vi "setup_oscillators.vi"(8 "error in (no error)":errorcluster, 11 "Handle In":T1 {"Handle" format="0x%08x"; "Conn" format="0x%08x"}) -> (0 "error out":errorcluster, 3 "Handle Out":T1 {"Handle" format="0x%08x"; "Conn" format="0x%08x"})   [LabVIEW 2019]
uses:
  Equipment/Zurich Instruments LabOne/Public/ziTypeHandle.ctl
  Instrument_Setup.vi
  Equipment/Zurich Instruments LabOne/Public/Configure/ziSetValueDouble.vi
  Equipment/Zurich Instruments LabOne/Zurich Instruments LabOne.lvlib
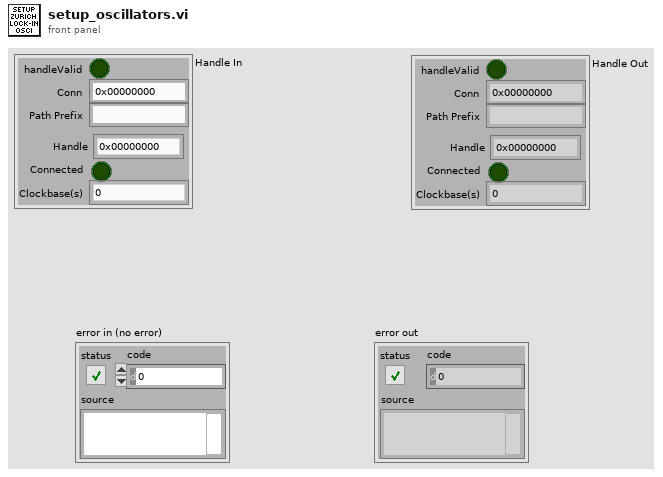
[diagram p1: front panel]
types:
  T1 = typedef "Zurich Instruments LabOne.lvlib/ziTypeHandle.ctl" = cluster{"handleValid":bool, "Conn":u64, "Path Prefix":string, "Handle":u64, "Connected":bool, "Clockbase(s)":dbl}
  T2 = typedef "Control 3.ctl" = cluster{"Adress":string, "Load Settings from File":bool, "Output_Demod1":enum16{"Aux 1", "Aux 2", "Aux 3", "Aux 4"}, "Input_Demod1":enum16{"Sig In 1", "Curr In 1", "Trigger 1", "Trigger 2", "Aux Out 1", "Aux Out 2", "Aux Out 3", "Aux Out 4", "Aux In 1", "Aux In 2", "Constant"}, "Input_Mode_Demod1":enum16{"single ended", "differential"}, "Bandwith_Mode_Demod1":enum16{"TC", "BW NEP", "BW 3dB"}, "Bandw_Value_demod1":dbl, "Demod1_Range":dbl, "Demod1_Harmonic":dbl, "Trigger_Demod1":enum16{"Manual", "External"}, "osc1_freq":dbl, "osc1_amp":dbl, "Demod1_scaling":dbl, "osc2_freq":dbl, "osc2_amp":dbl, "osc3_freq":dbl, "osc3_amp":dbl, "osc4_freq":dbl, "osc4_amp":dbl, "Demod1_Phase (deg)":dbl, "Demod1_order":ext, "Demod1_coupling":enum16{"DC", "AC"}, "Demod1_shields":enum16{"Ground", "Float"}, "Demod1_input_resistance":enum16{"10M", "50"}, "Demod1_Ref_oscillator":ext, "Demod1_output_imp":enum16{"Disable", "Enable"}, "Demod1_output_diff":enum16{"Disable", "Enable"}, "Demod1_rate":dbl, "Demod1_Output_range":dbl, "Output_Demod2":enum16{"Aux 1", "Aux 2", "Aux 3", "Aux 4"}, "Demod2_input":enum16{"Sig In 1", "Curr In 1", "Trigger 1", "Trigger 2", "Aux Out 1", "Aux Out 2", "Aux Out 3", "Aux Out 4", "Aux In 1", "Aux In 2", "Constant"}, "Input_Mode_Demod2":enum16{"single ended", "differential"}, "Bandwith_Mode_Demod2":enum16{"TC", "BW NEP", "BW 3dB"}, "Bandw_Value_demod2":dbl, "Demod2_Range":dbl, "Demod2_Harmonic":dbl, "Trigger_Demod2":enum16{"Manual", "External"}, "Demod2_scaling":dbl, "Demod2_Phase (deg)":dbl, "Demod2_order":ext, "Demod2_coupling":enum16{"DC", "AC"}, "Demod2_shields":enum16{"Ground", "Float"}, "Demod2_input_resistance":enum16{"10M", "50"}, "Demod2_Ref_oscillator":ext, "Demod2_output_imp":enum16{"Disable", "Enable"}, "Demod2_output_diff":enum16{"Disable", "Enable"}, "Demod2_rate":dbl, "Demod2_Output_range":dbl, "Output_Demod3":enum16{"Aux 1", "Aux 2", "Aux 3", "Aux 4"}, "Demod3_input":enum16{"Sig In 1", "Curr In 1", "Trigger 1", "Trigger 2", "Aux Out 1", "Aux Out 2", "Aux Out 3", "Aux Out 4", "Aux In 1", "Aux In 2", "Constant"}, "Input_Mode_Demod3":enum16{"single ended", "differential"}, "Bandwith_Mode_Demod2":enum16{"TC", "BW NEP", "BW 3dB"}, "Bandw_Value_demod3":dbl, "Demod3_Range":dbl, "Demod3_Harmonic":dbl, "Trigger_Demod3":enum16{"Manual", "External"}, "Demod3_scaling":dbl, "Demod3_Phase (deg)":dbl, "Demod3_order":ext, "Demod3_coupling":enum16{"DC", "AC"}, "Demod3_shields":enum16{"Ground", "Float"}, "Demod3_input_resistance":enum16{"10M", "50"}, "Demod3_Ref_oscillator":ext, "Demod3_output_imp":enum16{"Disable", "Enable"}, "Demod3_output_diff":enum16{"Disable", "Enable"}, "Demod3_rate":dbl, "Demod3_Output_range":dbl, "Output_Demod4":enum16{"Aux 1", "Aux 2", "Aux 3", "Aux 4"}, "Demod4_input":enum16{"Sig In 1", "Curr In 1", "Trigger 1", "Trigger 2", "Aux Out 1", "Aux Out 2", "Aux Out 3", "Aux Out 4", "Aux In 1", "Aux In 2", "Constant"}, "Input_Mode_Demod4":enum16{"single ended", "differential"}, "Bandwith_Mode_Demod4":enum16{"TC", "BW NEP", "BW 3dB"}, "Bandw_Value_demod4":dbl, "Demod4_Range":dbl, "Demod4_Harmonic":dbl, "Trigger_Demod4":enum16{"Manual", "External"}, "Demod4_scaling":dbl, "Demod4_Phase (deg)":dbl, "Demod4_order":ext, "Demod4_coupling":enum16{"DC", "AC"}, "Demod4_shields":enum16{"Ground", "Float"}, "Demod4_input_resistance":enum16{"10M", "50"}, "Demod4_Ref_oscillator":ext, "Demod4_output_imp":enum16{"Disable", "Enable"}, "Demod4_output_diff":enum16{"Disable", "Enable"}, "Demod4_rate":dbl, "Demod4_Output_range":dbl, "Oscillator1_Amp_units":enum16{"Vpk", "Vrms", "VdBm"}, "Oscillator4_Amp_units":enum16{"Vpk", "Vrms", "VdBm"}, "Oscillator2_Amp_units":enum16{"Vpk", "Vrms", "VdBm"}, "Oscillator3_Amp_units":enum16{"Vpk", "Vrms", "VdBm"}, "Demod1_sync_filter":enum16{"Disable", "Enable"}, "Demod 1 (on/off)":bool, "Demod 2 (on/off) ":bool, "Demod 3 (on/off) ":bool, "Demod 4 (on/off) ":bool, " Sigouts 1 (on/off)":bool, " Sigouts 2 (on/off) ":bool, " Sigouts 3 (on/off)":bool, " Sigouts 4 (on/off) ":bool, "Demod2_sync_filter":enum16{"Disable", "Enable"}, "Demod1_auto_outp_rang":enum16{"Disable", "Enable"}, "Demod2_auto_outp_rang ":enum16{"Disable", "Enable"}}
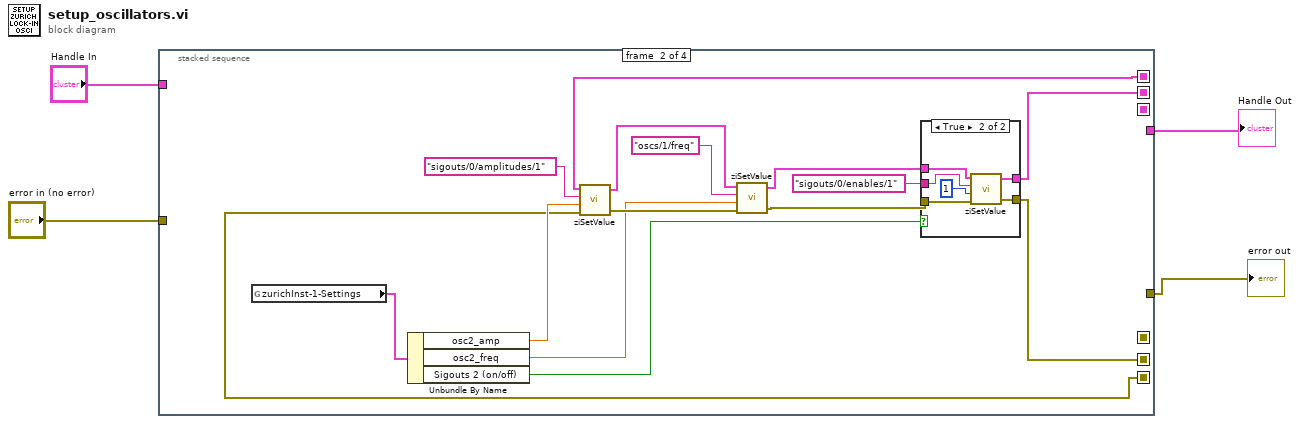
[diagram p0: block diagram]
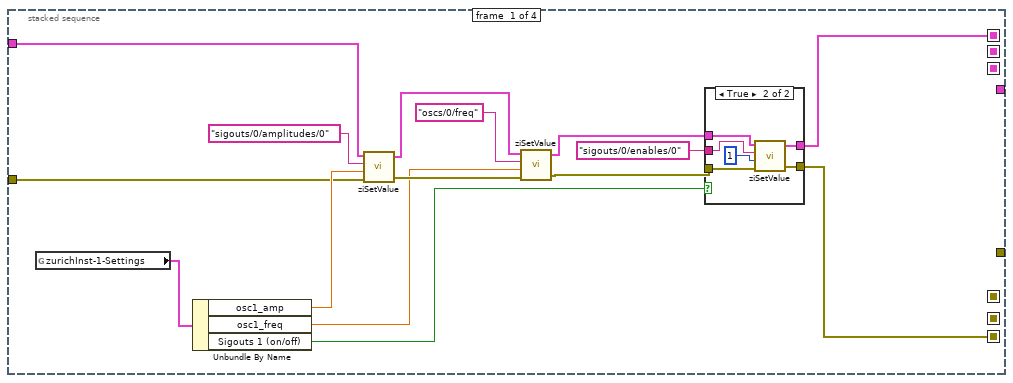
[diagram p2: hidden frame]
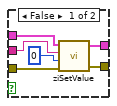
[diagram p3: hidden frame]
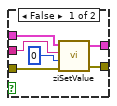
[diagram p4: hidden frame]
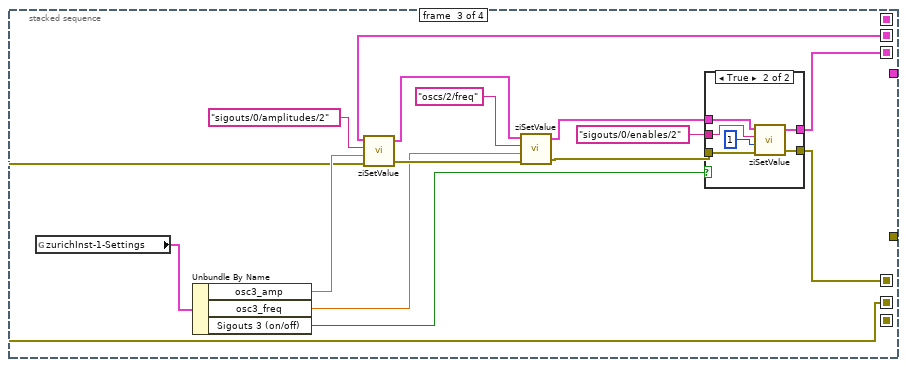
[diagram p5: hidden frame]
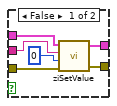
[diagram p6: hidden frame]
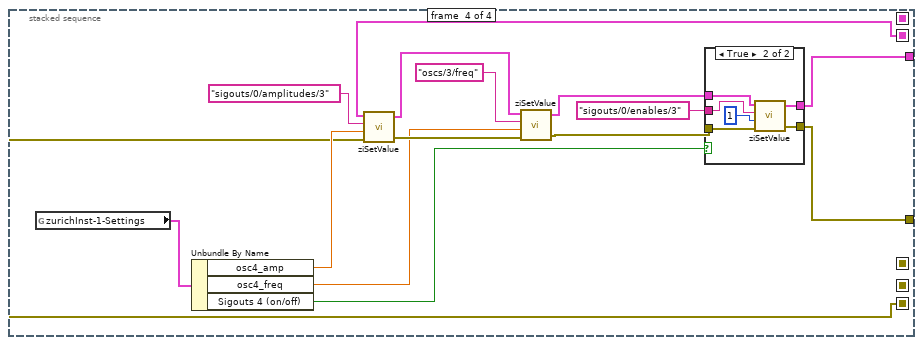
[diagram p7: hidden frame]
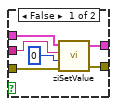
[diagram p8: hidden frame]
diagram:
  n1 = stacked-sequence {
    seq-local: [w7 _ _ _] -> [_ w32 _ w86]
    seq-local: [w5 _ _ _] -> [_ w35 _ _]
    seq-local: [_ w34 _ _] -> [_ _ w60 _]
    seq-local: [_ w33 _ _] -> [_ _ w62 _]
    seq-local: [_ _ w61 _] -> [_ _ _ _]
    seq-local: [_ _ w59 _] -> [_ _ _ w89]
    tunnel: "error in (no error)" -> [w8 _ _ _]
    tunnel: "Handle In" -> [w6 _ _ _]
    tunnel: [_ _ _ w88] -> w1
    tunnel: [_ _ _ w87] -> w2
    frame #0 {
      n2 = global read "Instrument_Setup.vi" "zurichInst-1-Settings"() -> (w18:T2)
      n3 = Unbundle By Name(w18) -> ("osc1_amp"=w15:dbl, "osc1_freq"=w13:dbl, "Sigouts 1 (on/off)"=w11:bool)
      n4 = call-poly "ziSetValue.vi"("Error In"=w8, "Value"=w15, "Path"="sigouts/0/amplitudes/0", "Handle In"=w6) -> ("Error Out"=w14:errorcluster, "Handle Out"=w16:T1)  [unwired: 1 in]
      n5 = call-poly "ziSetValue.vi"("Error In"=w14, "Value"=w13, "Path"="oscs/0/freq", "Handle In"=w16) -> ("Error Out"=w10:errorcluster, "Handle Out"=w9:T1)  [unwired: 1 in]
      n6 = case shown="True" w11 {
        tunnel: w10 -> [w23 w31]
        tunnel: w9 -> [w24 w30]
        tunnel: "sigouts/0/enables/0" -> [w25 w29]
        tunnel: [w20 w27] -> w5
        tunnel: [w21 w26] -> w7
        frame False {
          n7 = call-poly "ziSetValue.vi"("Error In"=w23, "Value"=0, "Path"=w25, "Handle In"=w24) -> ("Error Out"=w21:errorcluster, "Handle Out"=w20:T1)  [unwired: 1 in]
        }
        frame True {
          n8 = call-poly "ziSetValue.vi"("Error In"=w31, "Value"=1, "Path"=w29, "Handle In"=w30) -> ("Error Out"=w26:errorcluster, "Handle Out"=w27:T1)  [unwired: 1 in]
        }
      }
    }
    frame #1 {
      n9 = global read "Instrument_Setup.vi" "zurichInst-1-Settings"() -> (w45:T2)
      n10 = Unbundle By Name(w45) -> ("osc2_amp"=w42:dbl, "osc2_freq"=w40:dbl, "Sigouts 2 (on/off)"=w38:bool)
      n11 = call-poly "ziSetValue.vi"("Error In"=w32, "Value"=w42, "Path"="sigouts/0/amplitudes/1", "Handle In"=w35) -> ("Error Out"=w41:errorcluster, "Handle Out"=w43:T1)  [unwired: 1 in]
      n12 = call-poly "ziSetValue.vi"("Error In"=w41, "Value"=w40, "Path"="oscs/1/freq", "Handle In"=w43) -> ("Error Out"=w37:errorcluster, "Handle Out"=w36:T1)  [unwired: 1 in]
      n13 = case shown="True" w38 {
        tunnel: w37 -> [w50 w58]
        tunnel: w36 -> [w51 w57]
        tunnel: "sigouts/0/enables/1" -> [w52 w56]
        tunnel: [w47 w54] -> w34
        tunnel: [w48 w53] -> w33
        frame False {
          n14 = call-poly "ziSetValue.vi"("Error In"=w50, "Value"=0, "Path"=w52, "Handle In"=w51) -> ("Error Out"=w48:errorcluster, "Handle Out"=w47:T1)  [unwired: 1 in]
        }
        frame True {
          n15 = call-poly "ziSetValue.vi"("Error In"=w58, "Value"=1, "Path"=w56, "Handle In"=w57) -> ("Error Out"=w53:errorcluster, "Handle Out"=w54:T1)  [unwired: 1 in]
        }
      }
    }
    frame #2 {
      n16 = global read "Instrument_Setup.vi" "zurichInst-1-Settings"() -> (w72:T2)
      n17 = Unbundle By Name(w72) -> ("osc3_amp"=w69:dbl, "osc3_freq"=w67:dbl, "Sigouts 3 (on/off)"=w65:bool)
      n18 = call-poly "ziSetValue.vi"("Error In"=w62, "Value"=w69, "Path"="sigouts/0/amplitudes/2", "Handle In"=w60) -> ("Error Out"=w68:errorcluster, "Handle Out"=w70:T1)  [unwired: 1 in]
      n19 = call-poly "ziSetValue.vi"("Error In"=w68, "Value"=w67, "Path"="oscs/2/freq", "Handle In"=w70) -> ("Error Out"=w64:errorcluster, "Handle Out"=w63:T1)  [unwired: 1 in]
      n20 = case shown="True" w65 {
        tunnel: w64 -> [w77 w85]
        tunnel: w63 -> [w78 w84]
        tunnel: "sigouts/0/enables/2" -> [w79 w83]
        tunnel: [w74 w81] -> w59
        tunnel: [w75 w80] -> w61
        frame False {
          n21 = call-poly "ziSetValue.vi"("Error In"=w77, "Value"=0, "Path"=w79, "Handle In"=w78) -> ("Error Out"=w75:errorcluster, "Handle Out"=w74:T1)  [unwired: 1 in]
        }
        frame True {
          n22 = call-poly "ziSetValue.vi"("Error In"=w85, "Value"=1, "Path"=w83, "Handle In"=w84) -> ("Error Out"=w80:errorcluster, "Handle Out"=w81:T1)  [unwired: 1 in]
        }
      }
    }
    frame #3 {
      n23 = global read "Instrument_Setup.vi" "zurichInst-1-Settings"() -> (w99:T2)
      n24 = Unbundle By Name(w99) -> ("osc4_amp"=w96:dbl, "osc4_freq"=w94:dbl, "Sigouts 4 (on/off)"=w92:bool)
      n25 = call-poly "ziSetValue.vi"("Error In"=w86, "Value"=w96, "Path"="sigouts/0/amplitudes/3", "Handle In"=w89) -> ("Error Out"=w95:errorcluster, "Handle Out"=w97:T1)  [unwired: 1 in]
      n26 = call-poly "ziSetValue.vi"("Error In"=w95, "Value"=w94, "Path"="oscs/3/freq", "Handle In"=w97) -> ("Error Out"=w91:errorcluster, "Handle Out"=w90:T1)  [unwired: 1 in]
      n27 = case shown="True" w92 {
        tunnel: w91 -> [w104 w112]
        tunnel: w90 -> [w105 w111]
        tunnel: "sigouts/0/enables/3" -> [w106 w110]
        tunnel: [w101 w108] -> w88
        tunnel: [w102 w107] -> w87
        frame False {
          n28 = call-poly "ziSetValue.vi"("Error In"=w104, "Value"=0, "Path"=w106, "Handle In"=w105) -> ("Error Out"=w102:errorcluster, "Handle Out"=w101:T1)  [unwired: 1 in]
        }
        frame True {
          n29 = call-poly "ziSetValue.vi"("Error In"=w112, "Value"=1, "Path"=w110, "Handle In"=w111) -> ("Error Out"=w107:errorcluster, "Handle Out"=w108:T1)  [unwired: 1 in]
        }
      }
    }
  }
  "error out" <- w2
  "Handle Out" <- w1
